vi "Bottle_type.vi"(2 "Bottle assignments":T1, 4 "i":i32) -> (5 "active bottle index":i32, 6 "Bottle type":T2(ring))   [LabVIEW 2016]
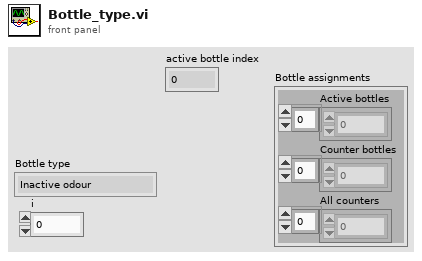
[diagram p1: front panel]
types:
  T1 = cluster{"Active bottles":i32[], "Counter bottles":i32[], "All counters":i32[]}
  T2 = enum16{"Inactive odour", "Active counter", "Inactive counter", "Active odour", "INVALID"}
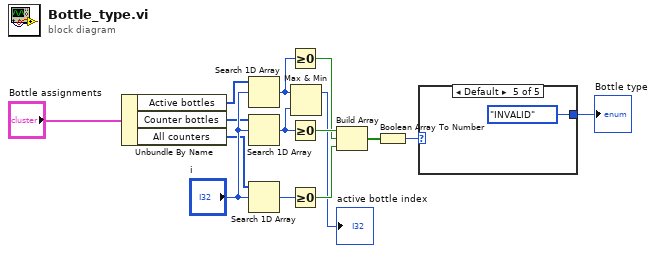
[diagram p0: block diagram]
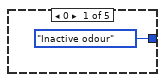
[diagram p2: hidden frame]
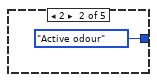
[diagram p3: hidden frame]
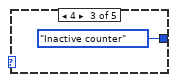
[diagram p4: hidden frame]
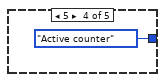
[diagram p5: hidden frame]
diagram:
  n1 = Unbundle By Name("Bottle assignments") -> ("Active bottles"=w6:i32[], "Counter bottles"=w5:i32[], "All counters"=w4:i32[])
  n2 = Search 1D Array(1D array=w6, element="i") -> (index of element=w3:i32)  [unwired: 1 in]
  n3 = Search 1D Array(1D array=w5, element="i") -> (index of element=w2:i32)  [unwired: 1 in]
  n4 = Search 1D Array(1D array=w4, element="i") -> (index of element=w14:i32)  [unwired: 1 in]
  n5 = Greater Or Equal To 0?(x=w3) -> (x >= 0?=w10:bool)
  n6 = Greater Or Equal To 0?(x=w2) -> (x >= 0?=w11:bool)
  n7 = Greater Or Equal To 0?(x=w14) -> (x >= 0?=w9:bool)
  n8 = Max & Min(x=w3, y=w2) -> (max(x,y)=→"active bottle index":i32)  [unwired: 1 out]
  n9 = Build Array(w11, w10, w9) -> (w8:bool[])
  n10 = Boolean Array To Number(Boolean array=w8) -> (number=w12:u32)
  n11 = case shown="Default" w12 {
    tunnel: [T2."Inactive odour" T2."Active odour" T2."Inactive counter" T2."Active counter" T2."INVALID"] -> w13
    frame 0 {
    }
    frame 2 {
    }
    frame 4 {
    }
    frame 5 {
    }
    frame Default {
    }
  }
  "Bottle type" <- w13
